vi "AODO-Engine.vi"(0 "Config":T2, 2 "Action":T5, 5 "AO":dbl[][](array[numeric]), 7 "DO":bool[][](array[boolean]), 11 "error in (no error)":errorcluster, 12 "Vmax":dbl[](array[numeric])) -> (4 "Config out":T2, 8 "Position":dbl, 10 "Sync Task":refnum<k21>, 14 "Tasks Out":T1[](array[typedef]), 15 "error out":errorcluster)   [LabVIEW 2020]
uses:
  Typedefs/AODO-Action.ctl
  Typedefs/AODO-Config.ctl
  Typedefs/AODO-Output Spec.ctl
  Typedefs/DO-Output Spec.ctl
  Typedefs/AODO-Task Specification.ctl
  <resource>/objmgr/daqmx.rc
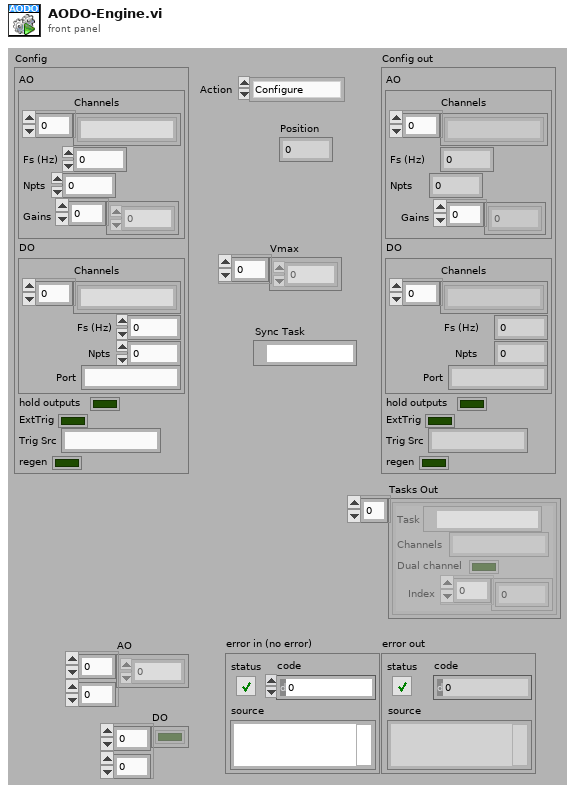
[diagram p1: front panel]
types:
  T1 = typedef "AODO-Task Specification.ctl" = cluster{"Task":refnum<k21>, "Channels":string, "Dual channel":bool, "Index":i32[]}
  T2 = typedef "AODO-Config.ctl" = cluster{"AO":T3, "DO":T4, "hold outputs":bool, "ExtTrig":bool, "Trig Src":string, "regen":bool}
  T3 = typedef "AODO-Output Spec.ctl" = cluster{"Channels":string[], "Fs (Hz)":dbl, "Npts":i32, "Gains":dbl[]}
  T4 = typedef "DO-Output Spec.ctl" = cluster{"Channels":string[], "Fs (Hz)":dbl, "Npts":i32, "Port":string}
  T5 = typedef "AODO-Action.ctl" = enum16{"Configure", "Initialize", "Start", "Write", "Clean up", "Init & Start", "Config & Test", "Position", "Set AO Gains", "Zero", "Prime"}
  T6 = typedef "AODO-DO Tasks.ctl" = cluster{"Active":bool, "clock task":refnum<k21>, "DO task":refnum<k21>}
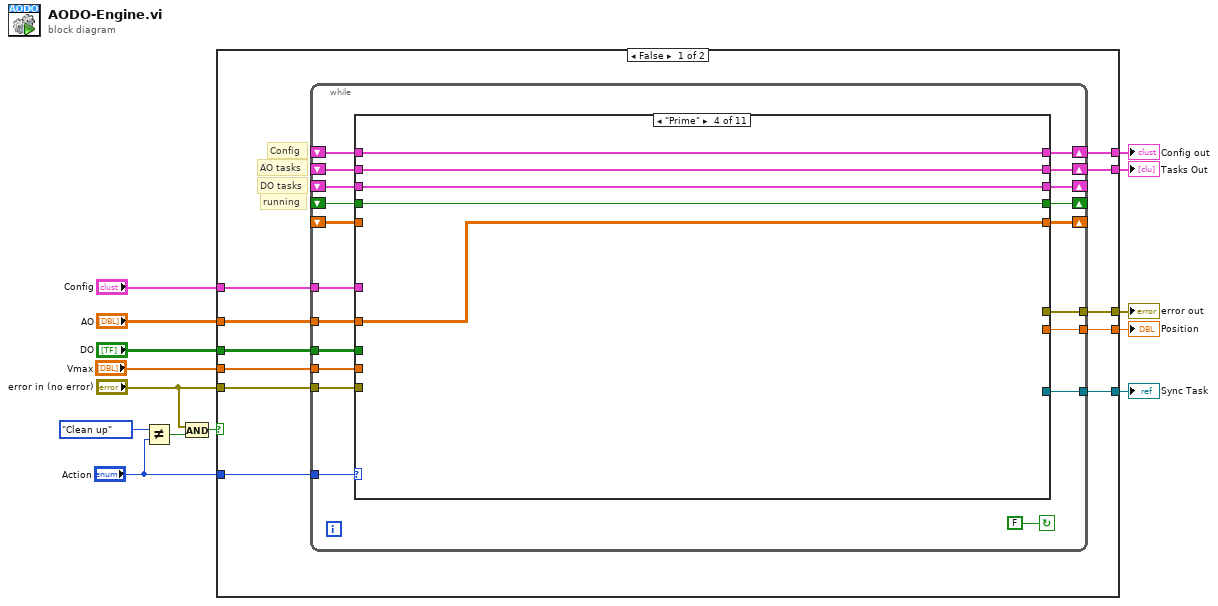
[diagram p0: block diagram]
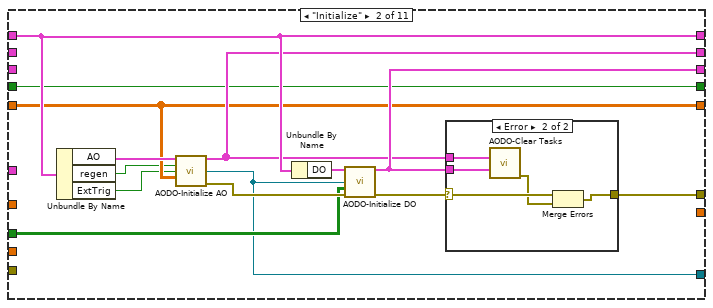
[diagram p3: hidden frame]
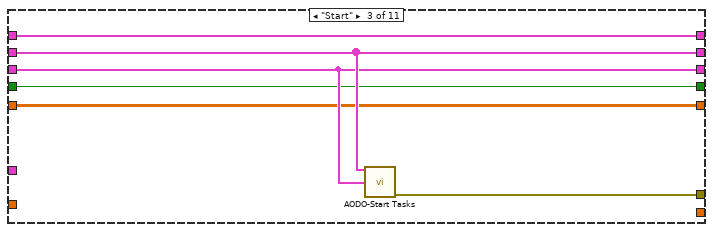
[diagram p5: hidden frame]
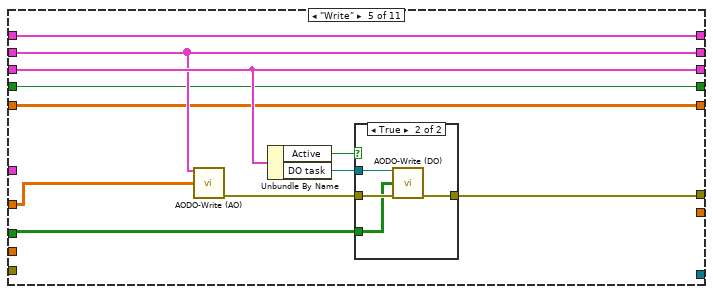
[diagram p6: hidden frame]
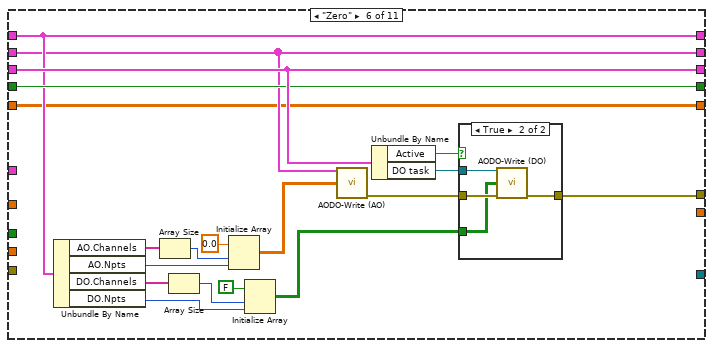
[diagram p8: hidden frame]
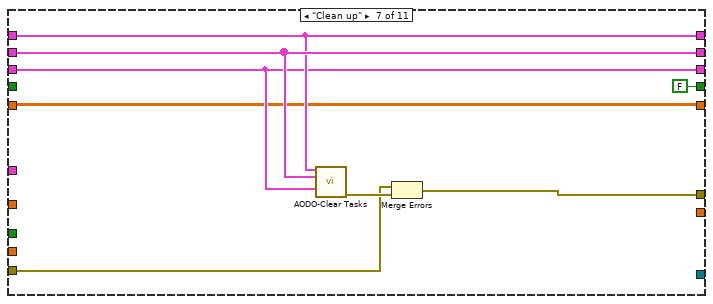
[diagram p10: hidden frame]
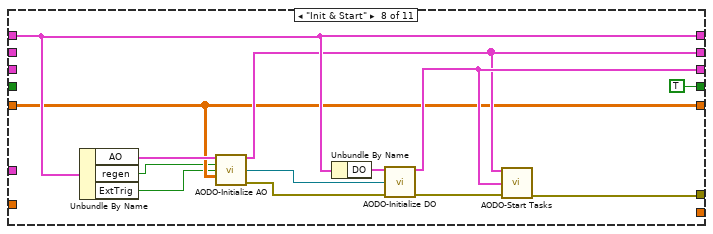
[diagram p11: hidden frame]
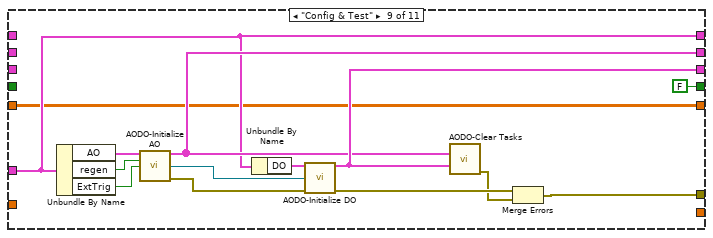
[diagram p12: hidden frame]
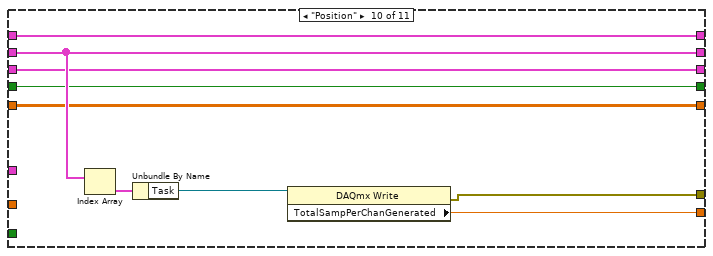
[diagram p13: hidden frame]
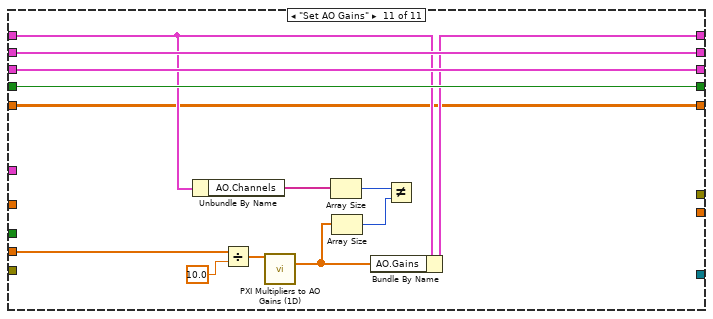
[diagram p14: hidden frame]
diagram:
  n1 = Not Equal?(x=AODO-Action."Clean up", y="Action") -> (x != y?=w8:bool)
  n2 = And(x="error in (no error)", y=w8) -> (x .and. y?=w9:bool)
  n3 = case shown="False" w9 {
    tunnel: "Action" -> [w25 _]
    tunnel: [w24 w179] -> w14
    tunnel: "Config" -> [w23 w178]
    tunnel: "AO" -> [w22 _]
    tunnel: "error in (no error)" -> [w18 w179]
    tunnel: "DO" -> [w21 _]
    tunnel: [w20 _] -> w5
    tunnel: "Vmax" -> [w19 _]
    tunnel: [w17 _] -> w3
    tunnel: [w16 w178] -> w2
    tunnel: [w15 _] -> w1
    frame False {
      # "running"
      # "Config"
      # "DO tasks"
      # "AO tasks"
      n4 = while {
        shift-right: [w37] -> w15
        shift-left: _ -> [w44]
        shift-right: [w43] -> _
        shift-left: _ -> [w42]
        tunnel: [w41] -> w24
        tunnel: w23 -> [w39]
        shift-right: [w40] -> w16
        shift-left: _ -> [w38]
        tunnel: w22 -> [w36]
        tunnel: w21 -> [w35]
        tunnel: w25 -> [w45]
        tunnel: [w33] -> w20
        shift-right: [w32] -> _
        shift-left: _ -> [w31]
        tunnel: w19 -> [w30]
        tunnel: w18 -> [w29]
        shift-right: [w28] -> _
        shift-left: _ -> [w27]
        tunnel: [w26] -> w17
        stop <- FALSE continue-if-true
        n5 = case shown="\"Prime\"" w45 {
          tunnel: [_ w57 w72 _ w82 w101 w123 w133 w148 w160 _] -> w41
          tunnel: w44 -> [w49 _ w74 w78 w84 w102 w127 _ _ w163 w175]
          tunnel: [w48 w59 w73 w80 w89 w115 w125 w135 w150 w157 w177] -> w43
          tunnel: w42 -> [w48 _ w73 w80 w89 w115 w125 _ _ w157 w177]
          tunnel: [w50 w61 w75 w79 w91 w113 w126 w137 w146 w164 w171] -> w40
          tunnel: w39 -> [w50 _ _ _ _ _ _ _ w146 _ _]
          tunnel: w38 -> [_ w61 w75 w79 w91 w113 w126 w137 _ w164 w169]
          tunnel: [w49 w58 w74 w78 w84 w102 w127 w134 w149 w163 w175] -> w37
          tunnel: w36 -> [w46 _ _ w76 w90 _ _ _ _ _ _]
          tunnel: w35 -> [_ w55 _ _ w85 _ _ _ _ _ _]
          tunnel: [_ _ _ _ _ _ _ _ _ w161 _] -> w33
          tunnel: [w47 w56 w71 w77 w83 w114 FALSE TRUE FALSE w158 w176] -> w32
          tunnel: w31 -> [w47 w56 w71 w77 w83 w114 _ _ _ w158 w176]
          tunnel: w30 -> [_ _ _ _ _ _ _ _ _ _ w174]
          tunnel: w29 -> [_ _ _ _ _ _ w122 _ _ _ _]
          tunnel: [w46 w54 w70 w76 w81 w97 w121 w131 w144 w156 w165] -> w28
          tunnel: w27 -> [_ w54 w70 _ w81 w97 w121 w131 w144 w156 w165]
          tunnel: [_ w53 _ _ _ _ _ _ _ _ _] -> w26
          frame "Configure", Default {
          }
          frame "Initialize" {
            n6 = Unbundle By Name(w61) -> ("AO"=w64:T3, "regen"=w52:bool, "ExtTrig"=w51:bool)
            n7 = call "AODO-Initialize AO.vi"("AO"=w64, "Regen?"=w52, "external trig"=w51, "AO data"=w54) -> ("Tasks Out"=w58:T1[], "Sync Task"=w53:refnum<k21>, "error out"=w63:errorcluster)  [unwired: 9 in]
            n8 = Unbundle By Name(w61) -> ("DO"=w62:T4)
            n9 = call "AODO-Initialize DO.vi"("DO"=w62, "Sync Task"=w53, "initialized array"=w55, "error in (no error)"=w63) -> ("DO Tasks"=w59:T6, "error out"=w60:errorcluster)  [unwired: 10 in]
            n10 = case shown="Error" w60 {
              selector: w60 -> [_ w68]
              tunnel: w59 -> [_ w65]
              tunnel: w58 -> [_ w69]
              tunnel: [_ w66] -> w57
              frame No Error {
              }
              frame Error {
                n11 = call "AODO-Clear Tasks.vi"("AO Tasks"=w69, "DO Tasks"=w65) -> ("error out"=w67:errorcluster)  [unwired: 13 in]
                n12 = Merge Errors(w68, w67) -> (w66:errorcluster)
              }
            }
          }
          frame "Start" {
            n13 = call "AODO-Start Tasks.vi"("AO Tasks"=w74, "DO Tasks"=w73) -> ("error out"=w72:errorcluster)  [unwired: 13 in]
          }
          frame "Prime" {
          }
          frame "Write" {
            n14 = call "AODO-Write (AO).vi"("Tasks In"=w84, "AO Waveforms"=w90) -> ("error out"=w87:errorcluster)  [unwired: 12 in, 1 out]
            n15 = Unbundle By Name(w89) -> ("Active"=w88:bool, "DO task"=w86:refnum<k21>)
            n16 = case shown="True" w88 {
              tunnel: w87 -> [w92 w95]
              tunnel: w86 -> [_ w96]
              tunnel: w85 -> [_ w94]
              tunnel: [w92 w93] -> w82
              frame False {
              }
              frame True {
                n17 = call "AODO-Write (DO).vi"("Task In"=w96, "DO Waveforms"=w94, "error in (no error)"=w95) -> ("error out"=w93:errorcluster)  [unwired: 11 in, 1 out]
              }
            }
          }
          frame "Zero" {
            n18 = Unbundle By Name(w113) -> ("AO.Channels"=w112:string[], "AO.Npts"=w110:i32, "DO.Channels"=w111:string[], "DO.Npts"=w106:i32)
            n19 = Array Size(array=w112) -> (size(s)=w109:i32)
            n20 = Array Size(array=w111) -> (size(s)=w105:i32)
            n21 = Initialize Array(0.0, w109, w110) -> (w107:dbl[][])
            n22 = Initialize Array(FALSE, w105, w106) -> (w103:bool[][])
            n23 = call "AODO-Write (AO).vi"("Tasks In"=w102, "AO Waveforms"=w107) -> ("error out"=w99:errorcluster)  [unwired: 12 in, 1 out]
            n24 = Unbundle By Name(w115) -> ("Active"=w100:bool, "DO task"=w98:refnum<k21>)
            n25 = case shown="True" w100 {
              tunnel: w99 -> [w116 w119]
              tunnel: w98 -> [_ w120]
              tunnel: w103 -> [_ w118]
              tunnel: [w116 w117] -> w101
              frame False {
              }
              frame True {
                n26 = call "AODO-Write (DO).vi"("Task In"=w120, "DO Waveforms"=w118, "error in (no error)"=w119) -> ("error out"=w117:errorcluster)  [unwired: 11 in, 1 out]
              }
            }
          }
          frame "Clean up" {
            n27 = call "AODO-Clear Tasks.vi"("Config"=w126, "AO Tasks"=w127, "DO Tasks"=w125) -> ("error out"=w128:errorcluster)  [unwired: 12 in]
            n28 = Merge Errors(w122, w128) -> (w123:errorcluster)
          }
          frame "Init & Start" {
            n29 = Unbundle By Name(w137) -> ("AO"=w141:T3, "regen"=w130:bool, "ExtTrig"=w129:bool)
            n30 = call "AODO-Initialize AO.vi"("AO"=w141, "Regen?"=w130, "external trig"=w129, "AO data"=w131) -> ("Tasks Out"=w134:T1[], "Sync Task"=w138:refnum<k21>, "error out"=w140:errorcluster)  [unwired: 9 in]
            n31 = Unbundle By Name(w137) -> ("DO"=w139:T4)
            n32 = call "AODO-Initialize DO.vi"("DO"=w139, "Sync Task"=w138, "error in (no error)"=w140) -> ("DO Tasks"=w135:T6, "error out"=w136:errorcluster)  [unwired: 11 in]
            n33 = call "AODO-Start Tasks.vi"("AO Tasks"=w134, "DO Tasks"=w135, "error in (no error)"=w136) -> ("error out"=w133:errorcluster)  [unwired: 12 in]
          }
          frame "Config & Test" {
            n34 = Unbundle By Name(w146) -> ("AO"=w155:T3, "regen"=w143:bool, "ExtTrig"=w142:bool)
            n35 = call "AODO-Initialize AO.vi"("AO"=w155, "Regen?"=w143, "external trig"=w142) -> ("Tasks Out"=w149:T1[], "Sync Task"=w152:refnum<k21>, "error out"=w154:errorcluster)  [unwired: 10 in]
            n36 = Unbundle By Name(w146) -> ("DO"=w153:T4)
            n37 = call "AODO-Initialize DO.vi"("DO"=w153, "Sync Task"=w152, "error in (no error)"=w154) -> ("DO Tasks"=w150:T6, "error out"=w151:errorcluster)  [unwired: 11 in]
            n38 = call "AODO-Clear Tasks.vi"("AO Tasks"=w149, "DO Tasks"=w150) -> ("error out"=w147:errorcluster)  [unwired: 13 in]
            n39 = Merge Errors(w151, w147) -> (w148:errorcluster)
          }
          frame "Position" {
            n40 = Index Array(array=w163) -> (element=w162:T1)  [unwired: 1 in]
            n41 = Unbundle By Name(w162) -> ("Task"=w159:refnum<k21>)
            n42 = property class="DAQmx Write"(reference=w159) -> (error out=w160:errorcluster, "TotalSampPerChanGenerated"=w161:dbl)  [unwired: 1 in, 1 out]
          }
          frame "Set AO Gains" {
            n43 = Unbundle By Name(w169) -> ("AO.Channels"=w168:string[])
            n44 = Divide(x=w174, y=10.0 ("Numeric")) -> (x/y=w173:dbl[])
            n45 = call "PXI Multipliers to AO Gains (1D).vi"("Multipliers in"=w173) -> ("Gains"=w170:dbl[])  [unwired: 12 in, 2 out]
            n46 = Array Size(array=w168) -> (size(s)=w167:i32)
            n47 = Array Size(array=w170) -> (size(s)=w166:i32)
            n48 = Bundle By Name(cluster=w169, "AO.Gains"=w170) -> (w171:T2)
            n49 = Not Equal?(x=w167, y=w166) -> ()  [unwired: 1 out]
          }
        }
      }
    }
    frame True {
    }
  }
  "error out" <- w14
  "Position" <- w5
  "Sync Task" <- w3
  "Config out" <- w2
  "Tasks Out" <- w1
